vi "New.vi"(8 "error in (no error)":errorcluster, 11 "reference in":refnum<class "TestCSMSuite.lvclass">) -> (0 "error out":errorcluster, 3 "reference out":refnum<class "TestCSMSuite.lvclass">)   [LabVIEW 2017, in "TestCSMSuite.lvclass"]
uses:
  TestCSMSuite.lvclass
  C:/Program Files (x86)/National Instruments/LabVIEW 2017/vi.lib/addons/_JKI Toolkits/VI Tester/TestSuite.llb/TestSuite.lvclass
  <vilib>/addons/_JKI Toolkits/VI Tester/TestCase.llb/TestCase.lvclass
  testcase-CSMMessage/testcase-CSMMessage.lvclass
  C:/Program Files (x86)/National Instruments/LabVIEW 2017/vi.lib/addons/_JKI Toolkits/VI Tester/TestCase.llb/TestCase.lvclass
  testcase-CSMArgument/testcase-CSMArgument.lvclass
  testcase-CSMResponse/testcase-CSMResponse.lvclass
  testcase-CSMGlobalLog/testcase-CSMGlobalLog.lvclass
  testcase-CSMStatus/testcase-CSMBroadcast.lvclass
  testcase-CSMSystemLevelModule/testcase-CSMSystemLevelModule.lvclass
  testcase-CSMSubModule/testcase-CSMSubModule.lvclass
  testcase-CSMWorkerMode/testcase-CSMWorkerMode.lvclass
  testcase-CSMChainMode/testcase-CSMChainMode.lvclass
  testcase-CSMChainMode/testcase-CSMManagementAPI/testcase-CSMManagementAPI.lvclass
  testcase-CSMNonCSMCallerSupportAPI/testcase-CSMNonCSMCallerSupportAPI.lvclass
  TestCSMSuite.lvclass/TestCSMSuite.ctl
  <vilib>/addons/_JKI Toolkits/VI Tester/TestSuite.llb/TestSuite.lvclass
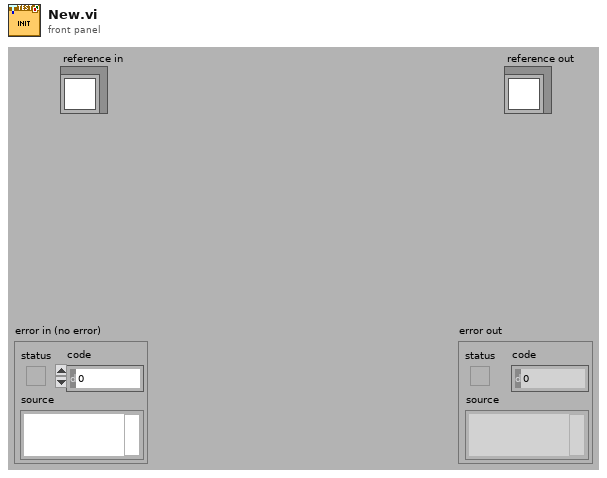
[diagram p1: front panel]
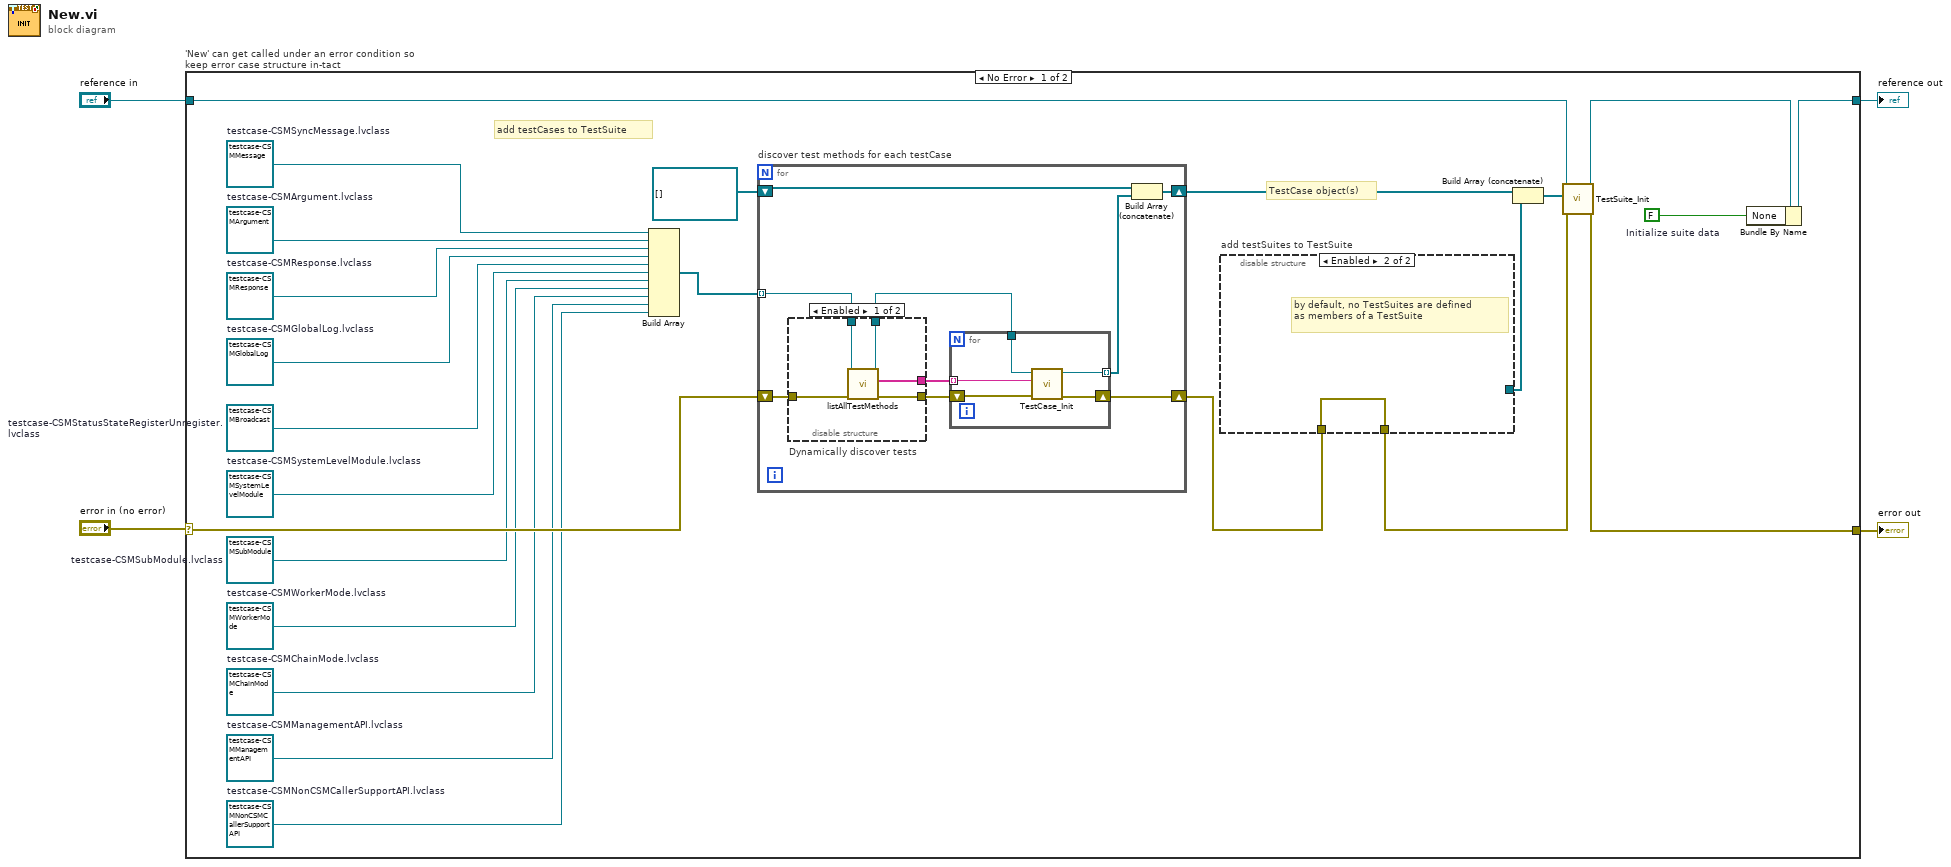
[diagram p0: block diagram]
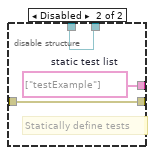
[diagram p2: hidden frame]
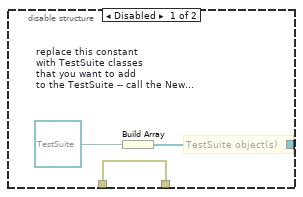
[diagram p3: hidden frame]
diagram:
  n1 = case "'New' can get called under an error condition so keep error case structure in-tact" shown="No Error" "error in (no error)" {
    selector: "error in (no error)" -> [w22 w55]
    tunnel: [w28 w56] -> w4
    tunnel: "reference in" -> [w23 w56]
    tunnel: [w25 w55] -> w1
    frame No Error {
      w5 = refnum<class "testcase-CSMNonCSMCallerSupportAPI.lvclass"> refnum  # testcase-CSMNonCSMCallerSupportAPI.lvclass
      w6 = refnum<class "testcase-CSMManagementAPI.lvclass"> refnum  # testcase-CSMManagementAPI.lvclass
      w7 = refnum<class "testcase-CSMChainMode.lvclass"> refnum  # testcase-CSMChainMode.lvclass
      w8 = refnum<class "testcase-CSMWorkerMode.lvclass"> refnum  # testcase-CSMWorkerMode.lvclass
      w9 = refnum<class "testcase-CSMSubModule.lvclass"> refnum  # testcase-CSMSubModule.lvclass
      w10 = refnum<class "testcase-CSMSystemLevelModule.lvclass"> refnum  # testcase-CSMSystemLevelModule.lvclass
      w11 = refnum<class "testcase-CSMBroadcast.lvclass"> refnum  # testcase-CSMStatusStateRegisterUnregister.lvclass
      w12 = refnum<class "testcase-CSMGlobalLog.lvclass"> refnum  # testcase-CSMGlobalLog.lvclass
      w13 = refnum<class "testcase-CSMResponse.lvclass"> refnum  # testcase-CSMResponse.lvclass
      w14 = refnum<class "testcase-CSMArgument.lvclass"> refnum  # testcase-CSMArgument.lvclass
      w15 = refnum<class "testcase-CSMMessage.lvclass"> refnum  # testcase-CSMSyncMessage.lvclass
      w27 = FALSE  # Initialize suite data
      # "TestCase object(s)"
      # "add testCases to TestSuite"
      n2 = Build Array(w15, w14, w13, w12, w11, w10, w9, w8, w7, w6, w5) -> (w24:refnum<class "TestCase.lvclass">[])
      n3 = for "discover test methods for each testCase" {
        shift-right: [w37] -> w17
        shift-left: w22 -> [w33]
        tunnel: w24 -> [w30] mode=indexing
        shift-right: [w34] -> w21
        shift-left: refnum<class "TestCase.lvclass">[] [] -> [w35]
        n4 = disable-structure "Dynamically discover tests" shown="Enabled" {
          disable-tunnel: w33 -> [w42 w43]
          disable-tunnel: [w41 w43] -> w32
          disable-tunnel: [w40 w44] -> w31
          disable-tunnel: w30 -> [w39 w45]
          disable-tunnel: [w38 w45] -> w29
          frame Enabled {
            n5 = call-dynamic "listAllTestMethods.vi"("error in (no error)"=w42, "TestCase in"=w39) -> ("error out"=w41:errorcluster, "test methods"=w40:string[], "TestCase out"=w38:refnum<class "TestCase.lvclass">)  [unwired: 7 in]
          }
          frame Disabled {
            w44 = string[] ["testExample"]  # static test list
            # "Statically define tests"
          }
        }
        n6 = for {
          tunnel: w29 -> [w46]
          tunnel: w31 -> [w50] mode=indexing
          shift-right: [w48] -> w37
          shift-left: w32 -> [w49]
          tunnel: [w47] -> w36 mode=indexing
          n7 = call <vilib>:"TestCase_Init.vi"("error in (no error)"=w49, "methodName (\"runTest\")"=w50, "TestCase in"=w46) -> ("error out"=w48:errorcluster, "TestCase out"=w47:refnum<class "TestCase.lvclass">)  [unwired: 7 in]
        }
        n8 = Build Array (concatenate)(w35, w36) -> (w34:refnum<class "TestCase.lvclass">[])
      }
      n9 = disable-structure "add testSuites to TestSuite" shown="Enabled" {
        disable-tunnel: [w51 _] -> w19
        disable-tunnel: [w53 w54] -> w18
        disable-tunnel: w17 -> [w53 w54]
        frame Disabled {
          w52 = refnum<class "TestSuite.lvclass"> refnum  # replace this constant with TestSuite classes that you want to add to the TestSuite -- call the New method for each TestSuite prior to adding it to this TestSuite
          # "TestSuite object(s)"
          n10 = Build Array(w52) -> (w51:refnum<class "TestSuite.lvclass">[])
        }
        frame Enabled {
          # "by default, no TestSuites are defined\nas members of a TestSuite"
        }
      }
      n11 = Build Array (concatenate)(w21, w19) -> (w20:refnum<class>[])
      n12 = call <vilib>:"TestSuite_Init.vi"("error in (no error)"=w18, "tests (none)"=w20, "TestSuite in"=w23) -> ("error out"=w25:errorcluster, "TestSuite out"=w26:refnum<class "TestCSMSuite.lvclass">)  [unwired: 7 in]
      n13 = Bundle By Name(cluster=w26, "None"=w27) -> (w28:refnum<class "TestCSMSuite.lvclass">)
    }
    frame Error {
    }
  }
  "reference out" <- w4
  "error out" <- w1
